vi "sort configured channels.vi"(8 "error in":errorcluster, 11 "shared memory editor node":refnum<class "module editor node.lvclass">) -> (0 "error out":errorcluster, 3 "shared memory editor node out":refnum<class "module editor node.lvclass">)   [LabVIEW 2014, in "Shared Memory editor node.lvclass"]
uses:
  Shared Memory editor node.lvclass
  <vilib>/NI/DCAF/Tag Editor Core/Configuration Editor/Classes/Module editor node/module editor node.lvclass
  module/configuration/Shared Memory configuration.lvclass
  <vilib>/NI/Configuration Framework/serializable configuration/NISE_CEF_serializable configuration.lvclass
  module/configuration/Shared Memory configuration.lvclass/Shared Memory configuration.ctl
  module/configuration/Read Lines.vi
  module/configuration/Write Lines.vi
  module/configuration/Get Line Name.vi
  module/configuration/Find Duplicate.vi
  <vilib>/Utility/error.llb/Error Cluster From Error Code.vi
  <vilib>/NI/Tag Bus Module Framework/channel/TBM channel.lvclass
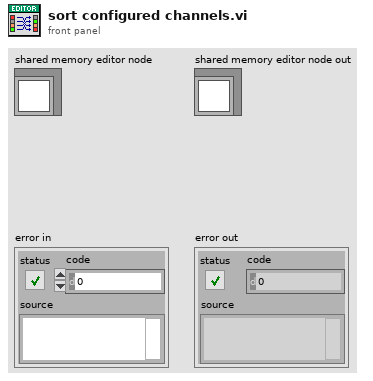
[diagram p1: front panel]
types:
  T1 = typedef "Shared Memory configuration.lvclass/Line.ctl" = cluster{"channel":refnum<class "TBM channel.lvclass">}
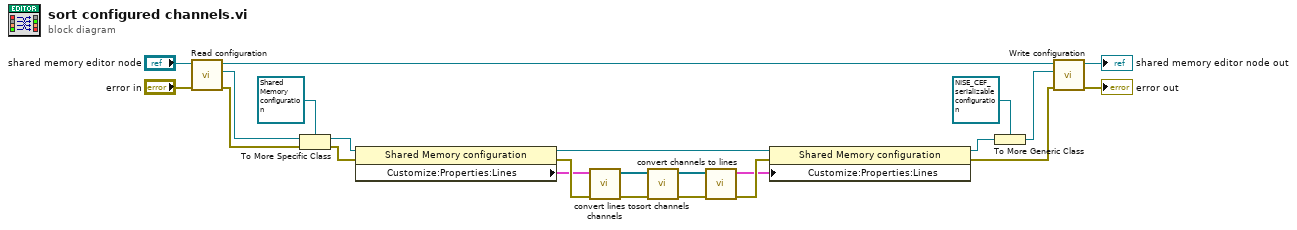
[diagram p0: block diagram]
diagram:
  n1 = call-dynamic "Read configuration.vi"("error in"="error in", "NISE_CEF_serializable node in"="shared memory editor node") -> ("error out"=w20:errorcluster, "configuration"=w21:refnum<class "NISE_CEF_serializable configuration.lvclass">, "NISE_CEF_serializable node out"=w15:refnum<class "module editor node.lvclass">)  [unwired: 7 in]
  n2 = To More Specific Class(target class=refnum<class "Shared Memory configuration.lvclass"> refnum ("shared memory configuration"), reference=w21, error in=w20) -> (specific class reference=w19:refnum<class "Shared Memory configuration.lvclass">, error out=w18:errorcluster)
  n3 = property class="Shared Memory configuration"(reference=w19, error in=w18) -> (reference out=w5:refnum<class "Shared Memory configuration.lvclass">, error out=w11:errorcluster, "Customize:Properties:Lines"=w10:T1[])
  n4 = call "convert lines to channels.vi"("error in (no error)"=w11, "Lines in"=w10) -> ("error out"=w9:errorcluster, "channels out"=w8:refnum<class "TBM channel.lvclass">[])  [unwired: 8 in]
  n5 = call "sort channels.vi"("error in (no error)"=w9, "channels in"=w8) -> ("error out"=w7:errorcluster, "channels out"=w6:refnum<class "TBM channel.lvclass">[])  [unwired: 8 in]
  n6 = call "convert channels to lines.vi"("error in (no error)"=w7, "channels"=w6) -> ("error out"=w4:errorcluster, "Lines"=w3:T1[])  [unwired: 8 in]
  n7 = property class="Shared Memory configuration"(reference=w5, error in=w4, "Customize:Properties:Lines"=w3) -> (reference out=w2:refnum<class "Shared Memory configuration.lvclass">, error out=w1:errorcluster)
  n8 = To More Generic Class(target class=refnum<class "NISE_CEF_serializable configuration.lvclass"> refnum ("configuration"), reference=w2) -> (generic class reference=w16:refnum<class "NISE_CEF_serializable configuration.lvclass">)
  n9 = call-dynamic "Write configuration.vi"("error in"=w1, "configuration"=w16, "NISE_CEF_serializable node in"=w15) -> ("error out"=→"error out":errorcluster, "NISE_CEF_serializable node out"=→"shared memory editor node out":refnum<class "module editor node.lvclass">)  [unwired: 7 in]
